vi "get control size.vi"(8 "error in (no error)":errorcluster, 11 "Control in":refnum<class "Path Control.lvclass">) -> (0 "error out":errorcluster, 2 "Size":T1, 3 "Control out":refnum<class "Path Control.lvclass">)   [LabVIEW 2010, in "Path Control.lvclass"]
uses:
  Path Control.lvclass
  <vilib>/Utility/miscctls.llb/LVBoundsTypeDef.ctl
  Control/Control.lvclass
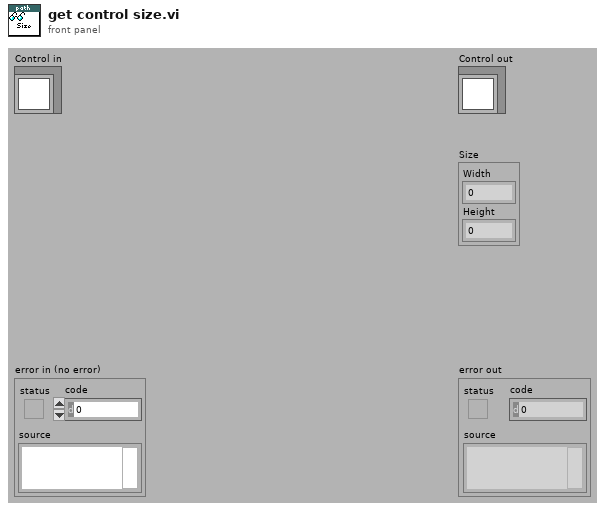
[diagram p1: front panel]
types:
  T1 = typedef "LVBoundsTypeDef.ctl" = cluster{"Width":u32, "Height":u32}
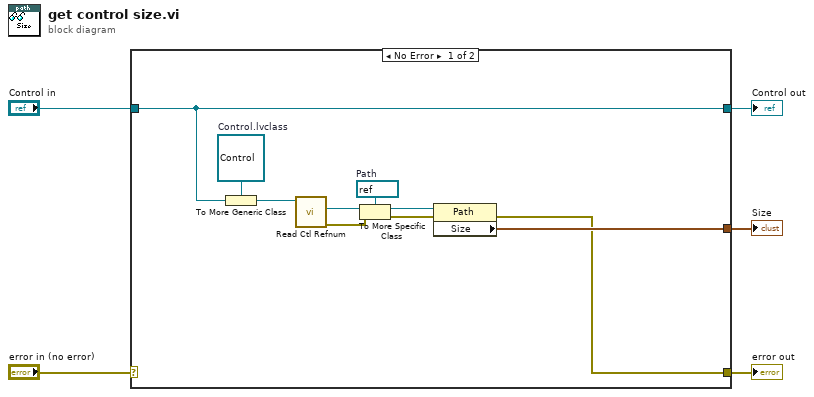
[diagram p0: block diagram]
diagram:
  n1 = case shown="No Error" "error in (no error)" {
    selector: "error in (no error)" -> [_ w17]
    tunnel: [w14 w17] -> w4
    tunnel: [w13 w16] -> w2
    tunnel: "Control in" -> [w13 w16]
    tunnel: [w15 _] -> w1
    frame No Error {
      w8 = refnum<vi> refnum  # Path
      w12 = refnum<class "Control.lvclass"> refnum  # Control.lvclass
      n2 = To More Generic Class(target class=w12, reference=w13) -> (generic class reference=w11:refnum<class "Control.lvclass">)
      n3 = call-dynamic "Read Ctl Refnum.vi"("Control in"=w11) -> ("error out"=w10:errorcluster, "Ctl Refnum"=w7:refnum<vi>)  [unwired: 8 in, 1 out]
      n4 = To More Specific Class(target class=w8, reference=w7, error in=w10) -> (specific class reference=w6:refnum<vi>, error out=w9:errorcluster)
      n5 = property class="Path"(reference=w6, error in=w9) -> (error out=w14:errorcluster, "Size"=w15:T1)  [unwired: 1 out]
    }
    frame Error {
    }
  }
  "error out" <- w4
  "Control out" <- w2
  "Size" <- w1
